vi "testLVPortCoreMatlab.vi"() -> ()   [LabVIEW 2017]
uses:
  Common/ObjectMap/LVPortObjectMapNamepathData.ctl
  Common/ObjectMap/LVPortObjectMapDataTypeEnum.ctl
  Common/ObjectMap/LVPortObjectMapContainerTypeEnum.ctl
panel:
  out "Updated":T1
  out "Matlab Param Data":T2[](array[typedef])
  in  "SomeDataType":T1
  out "pID":string
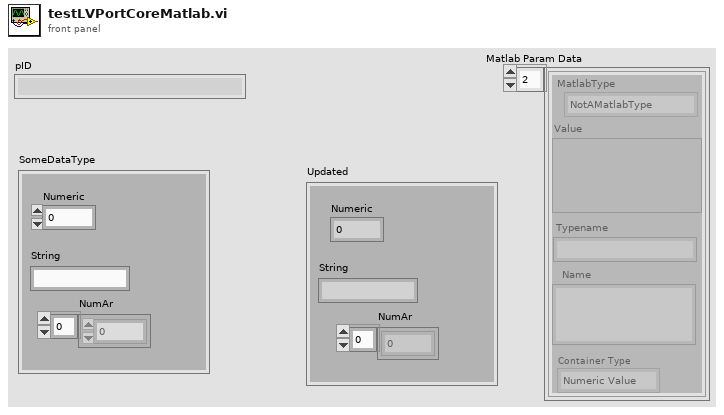
[diagram p1: front panel]
types:
  T1 = cluster{"Numeric":dbl, "String":string, "NumAr":dbl[]}
  T2 = typedef "LVPortObjectMapNamepathData.ctl" = cluster{"MatlabType":T3, "Value":variant, "Name":string, "Typename":string, "Container Type":T4}
  T3 = typedef "LVPortObjectMapDataTypeEnum.ctl" = enum16{"NotAMatlabType", "Real", "Complex", "String", "Boolean"}
  T4 = typedef "LVPortObjectMapContainerTypeEnum.ctl" = enum16{"Numeric Value", "Numeric Array", "Waveform"}
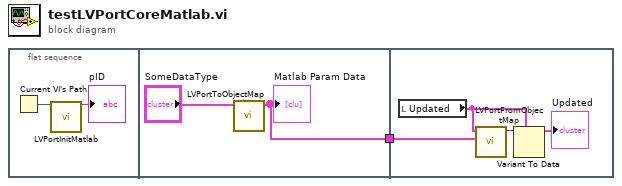
[diagram p0: block diagram]
diagram:
  n1 = flat-sequence {
    tunnel: [w4] -> w1
    tunnel: w1 -> [w9]
    frame #0 {
      n2 = Current VI's Path() -> (path=w3:path)
      n3 = call "LVPortInitMatlab.vi"("Working directory or VI Path"=w3) -> ("ID"=→"pID":string)  [unwired: 13 in, 1 out]
    }
    frame #1 {
      n4 = call "LVPortToObjectMap.vi"("Value"="SomeDataType") -> ("Matlab Param Data"=w4:T2[])  [unwired: 10 in]
      "Matlab Param Data" <- w4
    }
    frame #2 {
      n5 = local read "Updated"() -> (w7:T1)
      n6 = call "LVPortFromObjectMap.vi"("Matlab Param Data"=w9, "Type (or value to update)"=w7) -> ("Value"=w8:variant)  [unwired: 9 in]
      n7 = Variant To Data(type=w7, Variant=w8) -> (data=→"Updated":T1)  [unwired: 1 in, 1 out]
    }
  }
